vi "PID Line follower.vi"(4 "Port (Port 1)":T1=3 items=["Port 1", "Port 2", "Port 3", "Port 4"], 5 "K_d":sgl=16.0, 6 "K_i":sgl, 7 "K_p":sgl=0.3, 8 "Old Error":sgl, 9 "Previous integral":sgl, 10 "Target reflection":sgl, 11 "EV3 in":T2) -> (0 "New Error":sgl, 1 "New integral":sgl, 2 "Total error":sgl, 3 "EV3 out":T2)   [LabVIEW 2016]
uses:
  <vilib>/NXT/Subs/LVHSConnector.ctl
  <vilib>/NXT/LegoClasses/BrickReference/BrickReference.lvclass
  <vilib>/NXT/Block Support/NXT_InputPort.ctl
  <vilib>/NXT/Dual Mode Library/Sensors/EV3_Color_Reflect.vi
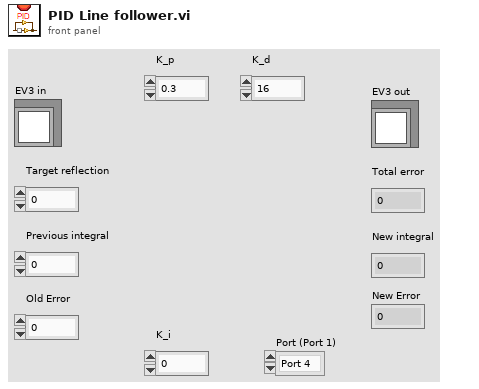
[diagram p1: front panel]
types:
  T1 = typedef "NXT_InputPort.ctl" = u32
  T2 = typedef "LVHSConnector.ctl" = refnum<class "BrickReference.lvclass">
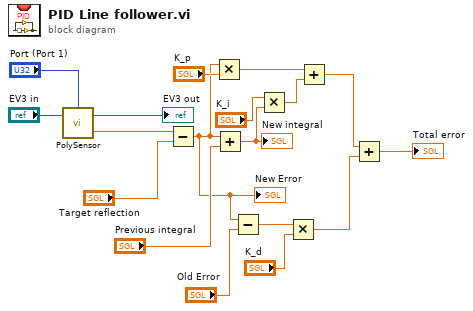
[diagram p0: block diagram]
diagram:
  n1 = call-poly <vilib>:"PolySensor.vi"("NXT/EV3"="EV3 in", "Port (Port 1)"="Port (Port 1)") -> ("Scaled Value"=w9:sgl, "NXT/EV3"=→"EV3 out":T2)  [unwired: 1 in]
  n2 = Subtract(x=w9, y="Target reflection") -> (x-y=w8:sgl)
  "New Error" <- w8
  n3 = Multiply(x=w8, y="K_p") -> (x*y=w14:sgl)
  n4 = Add(x=w8, y="Previous integral") -> (x+y=w12:sgl)
  "New integral" <- w12
  n5 = Subtract(x=w8, y="Old Error") -> (x-y=w6:sgl)
  n6 = Multiply(x="K_i", y=w12) -> (x*y=w15:sgl)
  n7 = Multiply(x=w6, y="K_d") -> (x*y=w4:sgl)
  n8 = Add(x=w14, y=w15) -> (x+y=w3:sgl)
  n9 = Add(x=w3, y=w4) -> (x+y=→"Total error":sgl)
